vi "Pasco Ready Shoot.vi"(9 "Light On/Locked On":bool, 10 "ShooterEncRate":dbl, 11 "ShooterDesRate":dbl) -> (3 "Feeder Output":dbl)   [LabVIEW 2011]
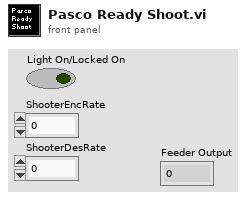
[diagram p1: front panel]
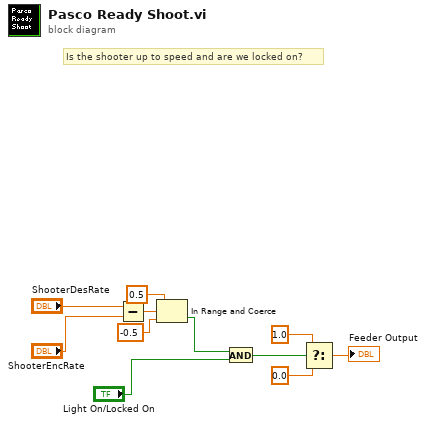
[diagram p0: block diagram]
diagram:
  # "Is the shooter up to speed and are we locked on?"
  n1 = Subtract(x="ShooterDesRate", y="ShooterEncRate") -> (x-y=w7:dbl)
  n2 = In Range and Coerce(upper limit=0.5, x=w7, lower limit=-0.5 ("upper limit")) -> (In Range?=w8:bool)  [unwired: 1 out]
  n3 = And(x=w8, y="Light On/Locked On") -> (x .and. y?=w9:bool)
  n4 = Select(t=1.0, s=w9, f=0.0) -> (s? t:f=→"Feeder Output":dbl)
